vi "Set Initialization Data - TCP Server.vi"(8 "error in":errorcluster, 11 "Head Worker in":refnum<class "Head Worker.lvclass">) -> (0 "error out":errorcluster, 3 "Head Worker out":refnum<class "Head Worker.lvclass">)   [LabVIEW 2017, in "Head Worker.lvclass"]
doc: "In this VI you can set the initialization data of a statically-linked subWorker."
uses:
  Head Worker.lvclass
  TCP Server/TCP Server/Initialization Data.ctl
  TCP Server/TCP Server/Response Cases.ctl
  <vilib>/addons/_Workers/Library/Case Label.ctl
  Head Worker.lvclass/Head Worker.ctl
  TCP Server/TCP Server/TCP Server.lvclass
  C:/Program Files (x86)/National Instruments/LabVIEW 2017/vi.lib/addons/_Workers/Library/Classes/Worker/Worker.lvclass
  <vilib>/addons/_Workers/Library/Workers.lvlib
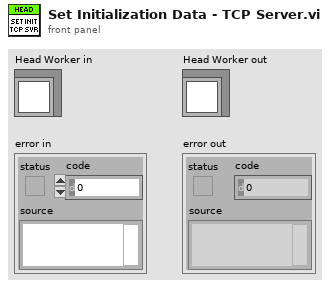
[diagram p1: front panel]
types:
  T1 = typedef "TCP Server.lvlib/TCP Server.lvclass/Initialization Data.ctl" = cluster{"Response Cases":T2}
  T2 = typedef "TCP Server.lvlib/TCP Server.lvclass/Response Cases.ctl" = cluster{"Incoming Data":T3, "Connection Notify":T3}
  T3 = typedef "Workers.lvlib/Case Label.ctl" = string
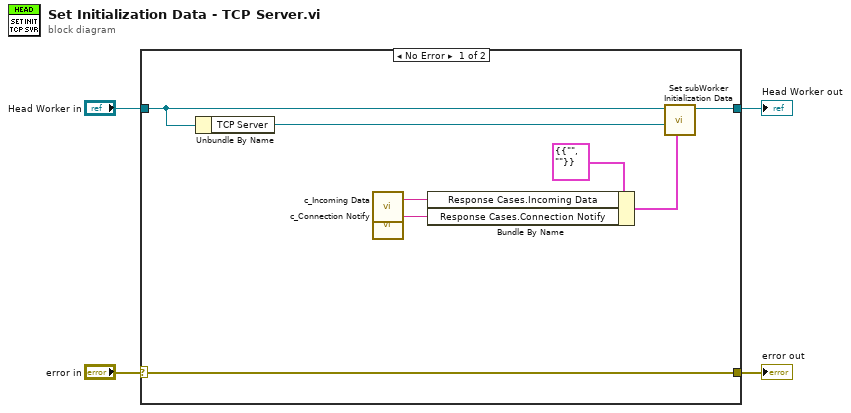
[diagram p0: block diagram]
diagram:
  n1 = case shown="No Error" "error in" {
    selector: "error in" -> [w12 w14]
    tunnel: [w12 w14] -> w3
    tunnel: [w10 w13] -> w2
    tunnel: "Head Worker in" -> [w9 w13]
    frame No Error {
      n2 = Unbundle By Name(w9) -> ("TCP Server"=w11:refnum<class "TCP Server.lvclass">)
      n3 = call "c_Incoming Data.vi"() -> ("Case Label"=w6:T3)  [unwired: 1 in]
      n4 = call "c_Connection Notify.vi"() -> ("Case Label"=w5:T3)  [unwired: 1 in]
      n5 = Bundle By Name(cluster=T1 {"Response Cases"={"Incoming Data"="", "Connection Notify"=""}} ("Initialization Data"), "Response Cases.Incoming Data"=w6, "Response Cases.Connection Notify"=w5) -> (w7:T1)
      n6 = call-dynamic "Set subWorker Initialization Data.vi"("Initialization Data"=w7, "subWorker"=w11, "Worker"=w9) -> ("Worker out"=w10:refnum<class "Head Worker.lvclass">)  [unwired: 8 in]
    }
    frame Error {
    }
  }
  "error out" <- w3
  "Head Worker out" <- w2
